vi "String to Data.vi"(7 "Len":u8, 8 "error in (no error)":errorcluster caption="错误输入（无错误）", 11 "String":string) -> (0 "error out":errorcluster caption="错误输出", 3 "Data":u8[](array[numeric]) format="%02x")   [LabVIEW 2018, in "CAN FD.lvlib"]
uses:
  CAN FD.lvlib
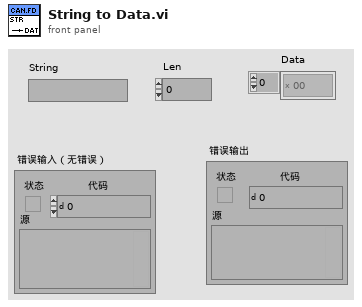
[diagram p1: front panel]
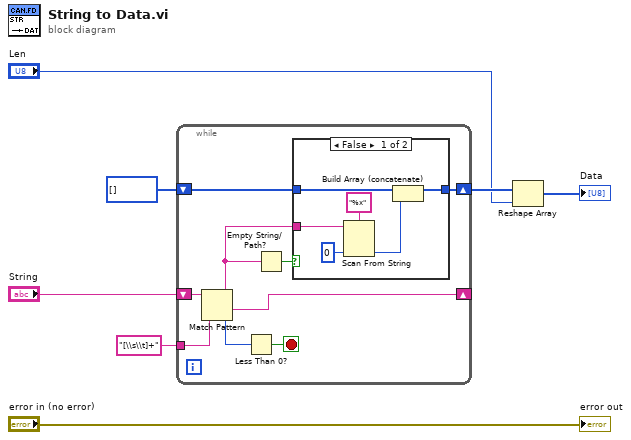
[diagram p0: block diagram]
diagram:
  n1 = while {
    shift-right: [w12] -> _
    shift-left: "String" -> [w16]
    tunnel: "[\\s\\t]+" -> [w15]
    shift-right: [w10] -> w3
    shift-left: u8[] [] -> [w9]
    stop <- w14 stop-if-true
    n2 = Match Pattern(string=w16, regular expression=w15) -> (before substring=w8:string, after substring=w12:string, offset past match=w13:i32)  [unwired: 1 in, 1 out]
    n3 = Less Than 0?(x=w13) -> (x < 0?=w14:bool)
    n4 = Empty String/Path?(string/path=w8) -> (empty?=w11:bool)
    n5 = case shown="False" w11 {
      tunnel: [w17 w23] -> w10
      tunnel: w9 -> [w19 w23]
      tunnel: w8 -> [w22 _]
      frame False {
        n6 = Scan From String(format string="%x" ("格式字符串"), input string=w22, default 1=u8 0 ("默认值 1")) -> (output 1=w18:u8)  [unwired: 2 in, 3 out]
        n7 = Build Array (concatenate)(w19, w18) -> (w17:u8[])
      }
      frame True {
      }
    }
  }
  n8 = Reshape Array(w3, "Len") -> (→"Data":u8[])
  "error out" <- "error in (no error)"
